vi "Main.vi"(11 "Module Admin":refnum<class "Delacor_lib_QMH_Module Admin.lvclass">) -> ()   [LabVIEW 2026, in "HMI.lvlib"]
doc: "This template is based off of the Queued Message Handler design pattern and the Queued Message Handler project template that ships with LabVIEW.\n\nThe main difference is that the queue is private to this module and communication between modules is performed via Broadcast and Request events.\n\nRequest events are wrapped in public API methods and are handled in the Event Handling Loop (EHL) of this VI. Any module can register for Broadcast events sent by this module. The EHL generates messages based on user interface actions.\n\nThe Message Handling Loop (MHL) processes messages generated by the EHL, or by other messages. The messages are string values, so new messages can be added easily to the Message Cases case structure in the MHL. Each message cluster can also provide an optional value for Message Data, which is a variant that can be converted to whatever message-specific data is required.\n_____\nBased on DQMH Dev Tools: Project Template 7.1.2.1547."
uses:
  HMI.lvlib
  <vilib>/Delacor/Delacor QMH/Libraries/Module Admin_class/Delacor_lib_QMH_Module Admin.lvclass
  Module Data--cluster.ctl
  <vilib>/Delacor/Delacor QMH/Libraries/Message Queue_class/Delacor_lib_QMH_Message Queue.lvclass/Delacor_lib_QMH_Message Queue.ctl
  Stop Argument--cluster.ctl
  <vilib>/Delacor/Delacor QMH/Libraries/Module Admin_class/Delacor_lib_QMH_Module Admin.lvclass/Delacor_lib_QMH_Module Admin.ctl
  <vilib>/Utility/miscctls.llb/LVPointTypeDef.ctl
  <vilib>/Delacor/Delacor QMH/Libraries/Message Queue_class/Delacor_lib_QMH_Enqueue Message (Single).vi
  <vilib>/Delacor/Delacor QMH/Libraries/Module Admin_class/Delacor_lib_QMH_Get External Launch.vi
  <vilib>/Delacor/Delacor QMH/Libraries/Message Queue_class/Delacor_lib_QMH_Message Queue.lvclass
  FT-818 CW Key Control/FT-818 CW Key Control.lvlib
  Plaintext to CW Sender/Plaintext to CW Sender.lvlib
panel:
  in  "CAT Rate":u32
  in  "Radio Comm Port":refnum<visa-resource-name>
  in  "Connect to FT-818":bool
  out "error out":errorcluster
  out "Status":string
  in  "Simulate MHL Error":bool
  in  "Simulate EHL Error":bool
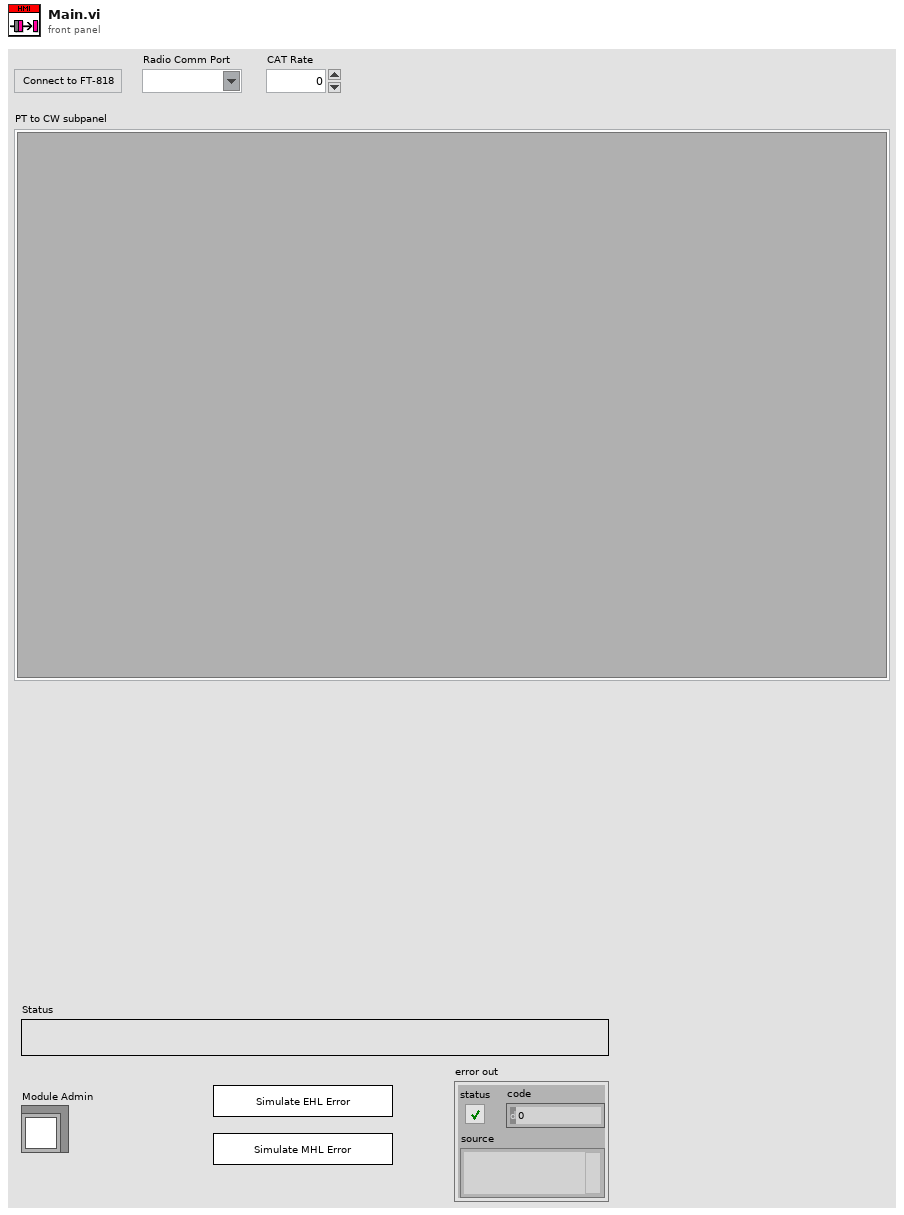
[diagram p1: front panel]
types:
  T1 = typedef "HMI.lvlib/Request Events--cluster.ctl" = cluster{"Stop Module":refnum<user-event>, "Show Panel":refnum<user-event>, "Hide Panel":refnum<user-event>, "Get Module Execution Status":refnum<user-event>, "Show Diagram":refnum<user-event>}
  T2 = typedef "FT-818 CW Key Control.lvlib/Broadcast Events--cluster.ctl" = cluster{"Module Did Init":refnum<user-event>, "Status Updated":refnum<user-event>, "Error Reported":refnum<user-event>, "Module Did Stop":refnum<user-event>, "Update Module Execution Status":refnum<user-event>}
  T3 = typedef "Plaintext to CW Sender.lvlib/Broadcast Events--cluster.ctl" = cluster{"Module Did Init":refnum<user-event>, "Status Updated":refnum<user-event>, "Error Reported":refnum<user-event>, "Module Did Stop":refnum<user-event>, "Update Module Execution Status":refnum<user-event>}
  T4 = typedef "HMI.lvlib/Module Data--cluster.ctl" = cluster{"Status":string}
  T5 = enum32{"invalid lock state", "Not Locked", "Locked (No Password)", "Password-protected"}
  T6 = typedef "HMI.lvlib/Stop Argument--cluster.ctl" = cluster{"Origin":string, "Exit via Stop Module Req?":bool, "Wait for Module to stop?":bool}
  T7 = typedef "LVPointTypeDef.ctl" = cluster{"Horizontal":i16, "Vertical":i16}
  T8 = enum32{"Invalid", "Standard", "Closed", "Hidden", "Minimized", "Maximized"}
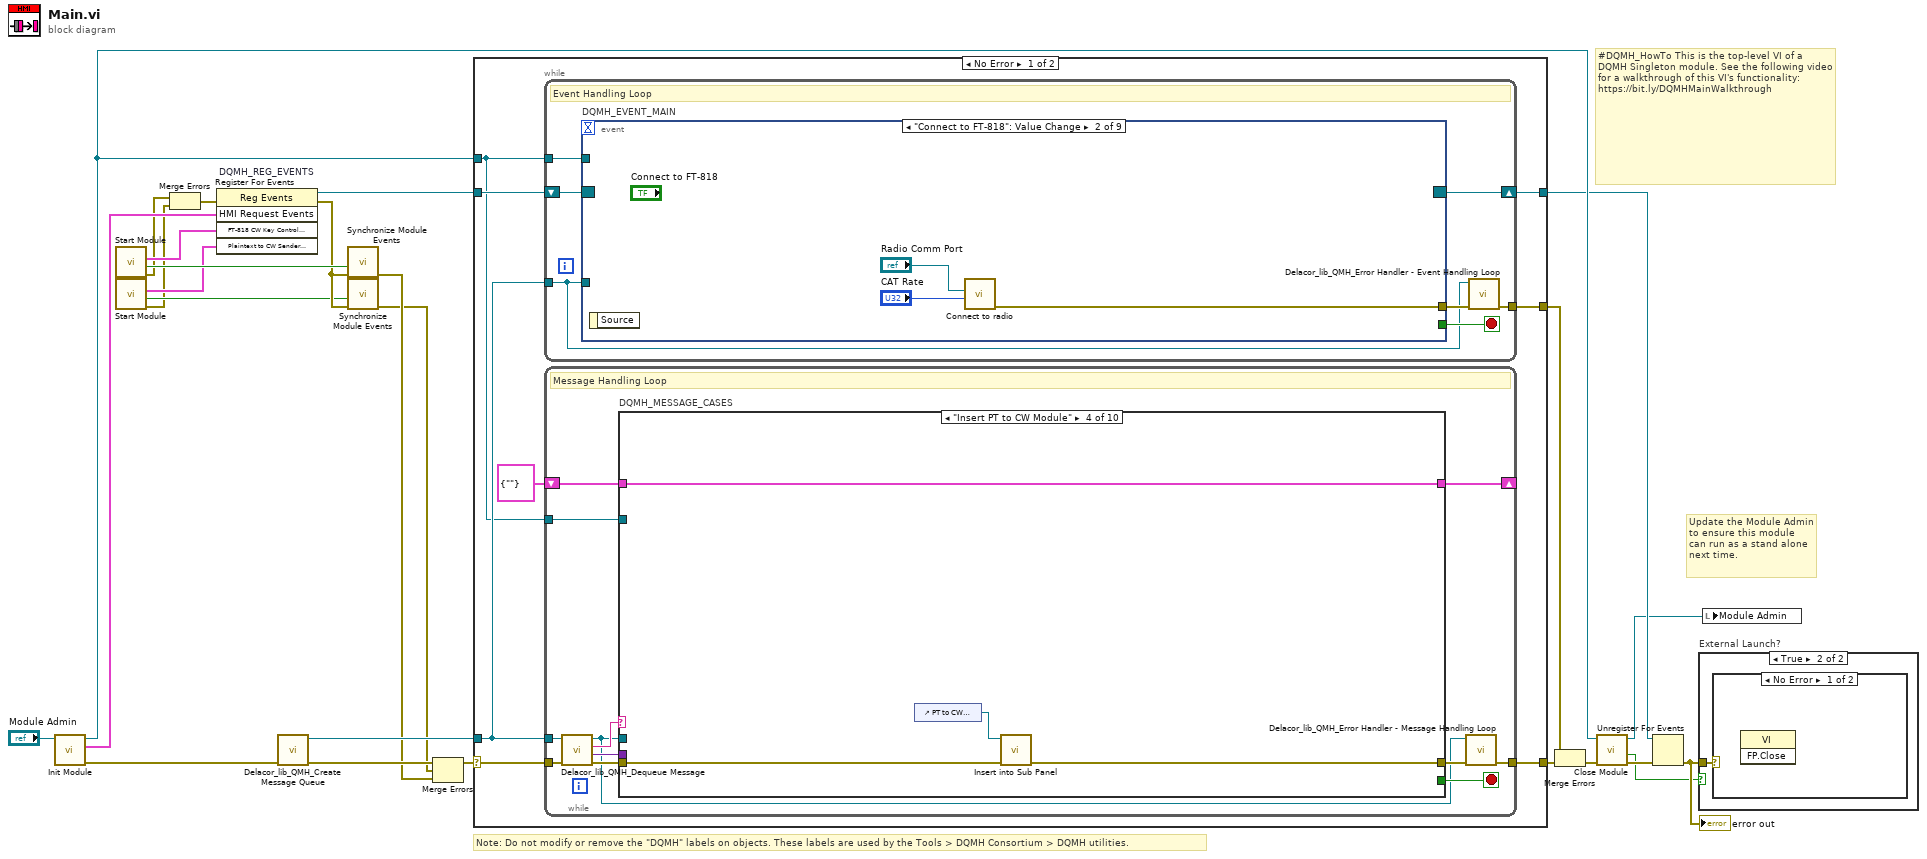
[diagram p0: block diagram]
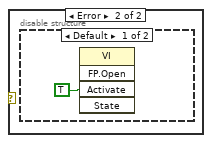
[diagram p3: hidden frame]
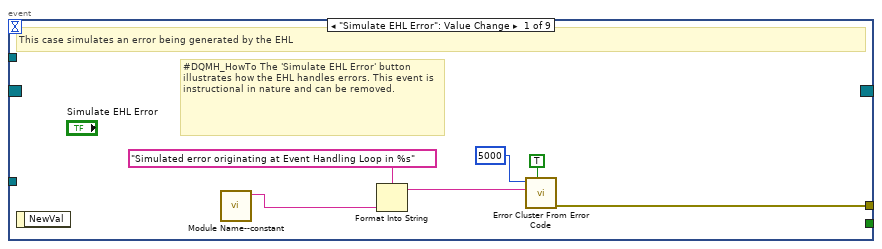
[diagram p5: hidden frame]
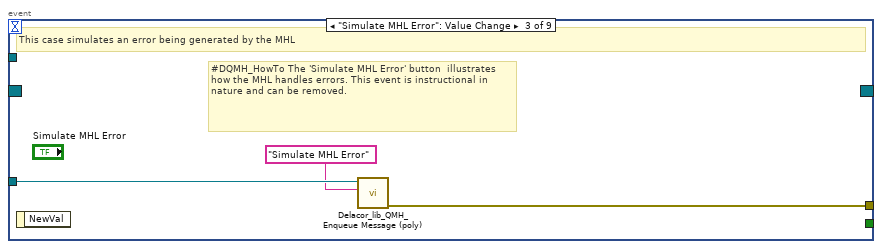
[diagram p6: hidden frame]
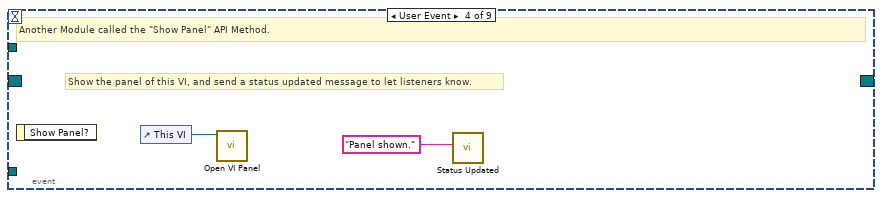
[diagram p7: hidden frame]
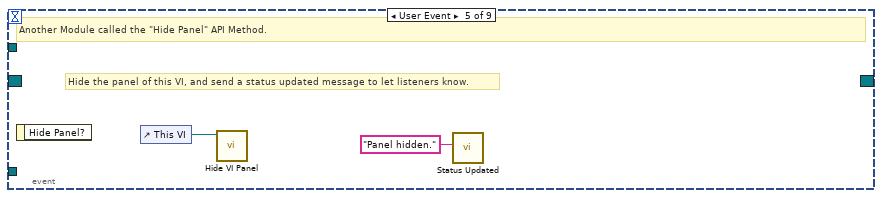
[diagram p8: hidden frame]
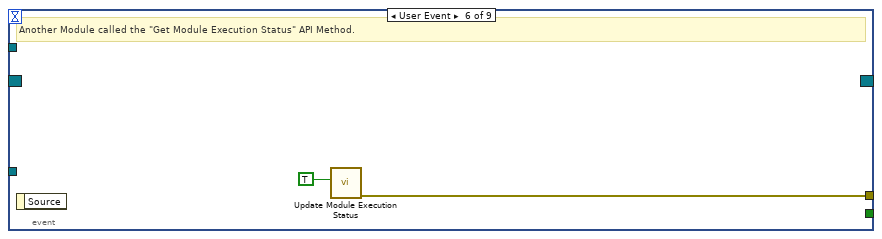
[diagram p9: hidden frame]
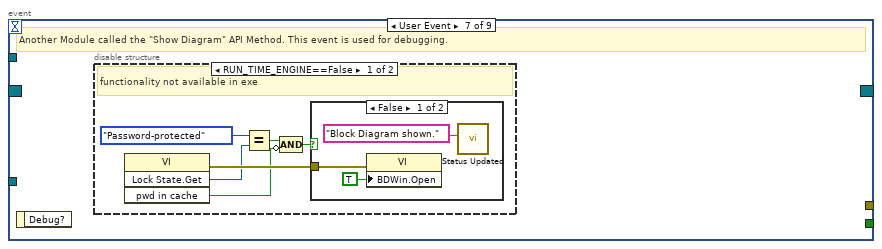
[diagram p10: hidden frame]
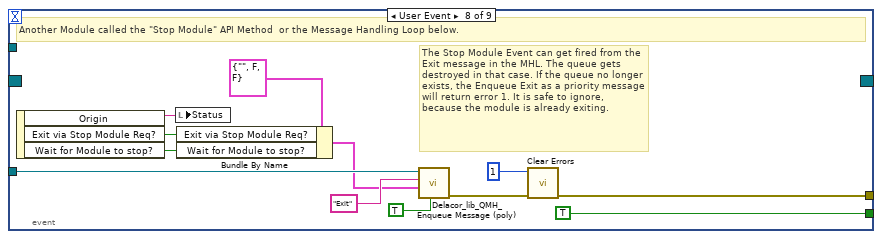
[diagram p13: hidden frame]
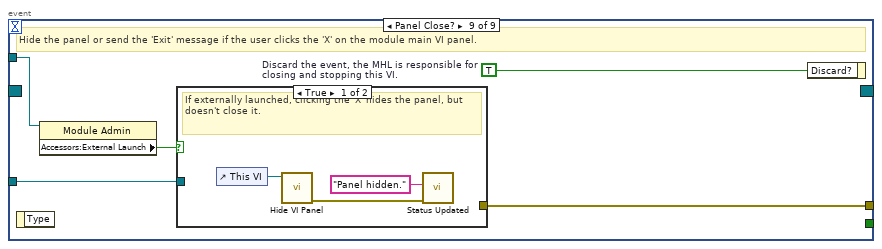
[diagram p14: hidden frame]
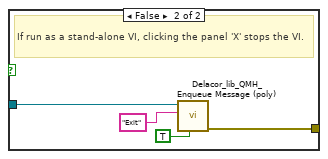
[diagram p15: hidden frame]
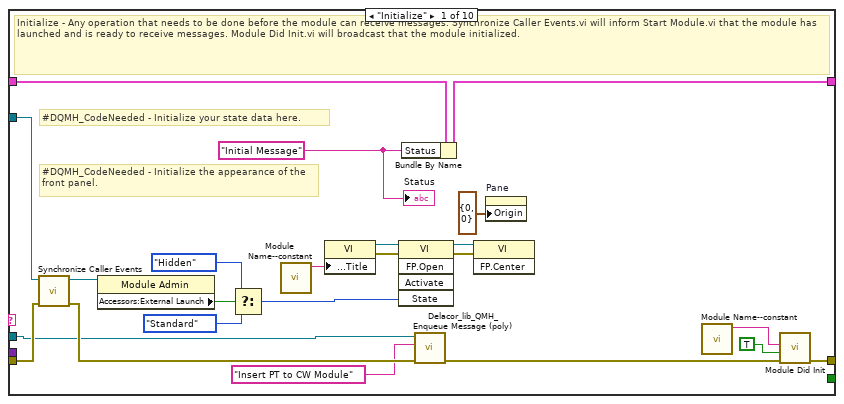
[diagram p16: hidden frame]
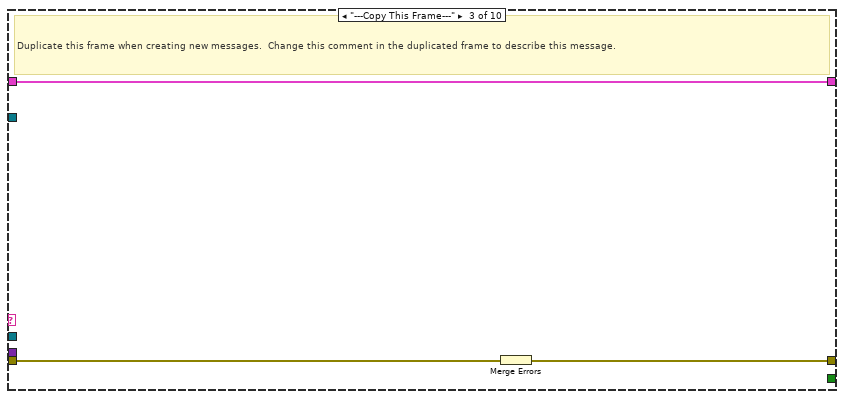
[diagram p18: hidden frame]
diagram:
  # "#DQMH_HowTo This is the top-level VI of a DQMH Singleton module. See the following video for a walkthrough of this VI's functionality: https://bit.ly/DQMHMainWalkthrough"
  # "Note: Do not modify or remove the \"DQMH\" labels on objects. These labels are used by the Tools > DQMH Consortium > DQMH utilities."
  # "Update the Module Admin to ensure this module can run as a stand alone next time."
  n1 = call "Init Module.vi"("Singleton Module Admin in"="Module Admin") -> ("error out"=w25:errorcluster, "HMI Request Events"=w15:T1, "Singleton Module Admin out"=w18:refnum<class "Delacor_lib_QMH_Module Admin.lvclass">)  [unwired: 8 in]
  n2 = call "Start Module.vi"() -> ("error out"=w3:errorcluster, "Wait for Event Sync?"=w9:bool, "FT-818 CW Key Control Broadcast Events"=w10:T2)  [unwired: 7 in, 2 out]
  n3 = call "Start Module.vi"() -> ("error out"=w2:errorcluster, "Wait for Event Sync?"=w4:bool, "Plaintext to CW Sender Broadcast Events"=w7:T3)  [unwired: 7 in, 2 out]
  n4 = Merge Errors(w3, w2) -> (w1:errorcluster)
  n5 = register-events "DQMH_REG_EVENTS"(error in=w1, w15, w10, w7) -> (reference out=w16:refnum<event-registration>, error out=w6:errorcluster)  [unwired: 1 in]
  n6 = call <vilib>:"Delacor_lib_QMH_Create Message Queue.vi"("error in"=w25) -> ("error out"=w20:errorcluster, "Message Queue"=w14:refnum<class "Delacor_lib_QMH_Message Queue.lvclass">)  [unwired: 9 in]
  n7 = call "Synchronize Module Events.vi"("error in"=w6, "Wait for Event Sync?"=w9) -> ("error out"=w8:errorcluster)  [unwired: 9 in]
  n8 = call "Synchronize Module Events.vi"("error in"=w6, "Wait for Event Sync?"=w4) -> ("error out"=w5:errorcluster)  [unwired: 9 in]
  n9 = Merge Errors(w20, w5, w8) -> (w19:errorcluster)
  n10 = case shown="No Error" w19 {
    selector: w19 -> [w32 w203]
    tunnel: [w34 w202] -> w26
    tunnel: [w31 w201] -> w17
    tunnel: w16 -> [w29 w201]
    tunnel: w14 -> [w28 w196]
    tunnel: [w33 _] -> w23
    tunnel: w18 -> [w27 w197]
    frame No Error {
      n11 = while {
        tunnel: w28 -> [w35]
        shift-right: [w38] -> w31
        shift-left: w29 -> [w39]
        tunnel: [w40] -> w33
        tunnel: w27 -> [w36]
        stop <- w37 stop-if-true
        # "Event Handling Loop"
        n12 = event "DQMH_EVENT_MAIN" shown="[1] \"Connect to FT-818\": Value Change" {
          selector: w39 -> [_ _ _ _ _ _ _ _ _]
          dyn-events: [_ _ _ _ _ _ _ _ _] -> w38
          timeout: _ -> [_ _ _ _ _ _ _ _ _]
          tunnel: [_ _ _ _ _ _ _ TRUE ("Discard?") _] -> w37
          tunnel: w35 -> [_ _ w52 _ _ _ _ w76 w83]
          tunnel: [w47 w50 w53 _ _ w59 _ w79 w85] -> w41
          tunnel: w36 -> [_ _ _ _ _ _ _ _ w82]
          event "Simulate EHL Error": Value Change {
            # "#DQMH_HowTo The 'Simulate EHL Error' button  illustrates how the EHL handles errors. This event is instructional in nature and can be removed."
            # "This case simulates an error being generated by the EHL"
            n13 = event-data() -> ()  [unwired: 1 in, 1 out]
            n14 = call "Module Name--constant.vi"() -> ("Module Name"=w44:string)  [unwired: 11 in]
            n15 = Format Into String(format string="Simulated error originating at Event Handling Loop in %s", w44) -> (resulting string=w45:string)  [unwired: 2 in, 1 out]
            n16 = call <vilib>:"Error Cluster From Error Code.vi"("show call chain? (False)"=TRUE, "error message (\"\")"=w45, "error code (0)"=5000) -> ("error out"=w47:errorcluster)  [unwired: 6 in]
          }
          event "Connect to FT-818": Value Change {
            n17 = event-data() -> ()  [unwired: 1 in, 1 out]
            n18 = call "Connect to radio.vi"("CAT Rate"="CAT Rate", "Radio Comm Port"="Radio Comm Port") -> ("error out"=w50:errorcluster)  [unwired: 7 in, 2 out]
          }
          event "Simulate MHL Error": Value Change {
            # "#DQMH_HowTo The 'Simulate MHL Error' button  illustrates how the MHL handles errors. This event is instructional in nature and can be removed."
            # "This case simulates an error being generated by the MHL"
            n19 = event-data() -> ()  [unwired: 1 in, 1 out]
            n20 = call-poly <vilib>:"Delacor_lib_QMH_Enqueue Message (poly).vi"("Message"="Simulate MHL Error", "Message Queue in"=w52) -> ("error out"=w53:errorcluster)  [unwired: 8 in, 1 out]
          }
          event User Event {
            # "Show the panel of this VI, and send a status updated message to let listeners know."
            # "Another Module called the \"Show Panel\" API Method."
            n21 = event-data() -> ()  [unwired: 1 in, 1 out]
            n22 = control-ref of="This VI"() -> (w55:refnum<vi>)
            n23 = call "Open VI Panel.vi"("VI"=w55) -> ()  [unwired: 10 in, 1 out]
            n24 = call "Status Updated.vi"("Status"="Panel shown." ("format string")) -> ()  [unwired: 10 in, 1 out]
          }
          event User Event {
            # "Hide the panel of this VI, and send a status updated message to let listeners know."
            # "Another Module called the \"Hide Panel\" API Method."
            n25 = event-data() -> ()  [unwired: 1 in, 1 out]
            n26 = control-ref of="This VI"() -> (w57:refnum<vi>)
            n27 = call "Hide VI Panel.vi"("VI"=w57) -> ()  [unwired: 10 in, 1 out]
            n28 = call "Status Updated.vi"("Status"="Panel hidden." ("format string")) -> ()  [unwired: 10 in, 1 out]
          }
          event User Event {
            # "Another Module called the \"Get Module Execution Status\" API Method."
            n29 = event-data() -> ()  [unwired: 1 in, 1 out]
            n30 = call "Update Module Execution Status.vi"("Running?"=TRUE) -> ("error out"=w59:errorcluster)  [unwired: 10 in]
          }
          event User Event {
            # "Another Module called the \"Show Diagram\" API Method. This event is used for debugging."
            n31 = event-data() -> ()  [unwired: 1 in, 1 out]
            n32 = disable-structure shown="RUN_TIME_ENGINE==False" {
              frame condition #0 (active) {
                # "functionality not available in exe"
                n33 = invoke on="Invoke Node" class="VI" method="Lock State.Get"() -> (error out=w65:errorcluster, "Get Lock State"=w64:T5, "pwd in cache"=w61:bool)  [unwired: 4 in, 1 out]
                n34 = Equal?(x=T5."Password-protected", y=w64) -> (x = y?=w62:bool)
                n35 = Compound Arithmetic op=AND(w62, invert w61) -> (w60:bool)
                n36 = case shown="False" w60 {
                  tunnel: w65 -> [w68 _]
                  frame False {
                    n37 = property on="Property Node" class="VI"(error in=w68, "BDWin.Open"=TRUE ("Block Diagram Window:Open")) -> ()  [unwired: 1 in, 2 out]
                    n38 = call "Status Updated.vi"("Status"="Block Diagram shown." ("format string")) -> ()  [unwired: 10 in, 1 out]
                  }
                  frame True {
                    # "Password-protected VI, and the password is not in the cache. Do not show the diagram."
                  }
                }
              }
              frame condition #1 {
              }
            }
          }
          event User Event {
            # "The Stop Module Event can get fired from the Exit message in the MHL. The queue gets destroyed in that case. If the queue no longer exists, the Enqueue Exit as a priority message will return error 1. It is safe to ignore, because the module is already exiting."
            # "Another Module called the \"Stop Module\" API Method  or the Message Handling Loop below."
            n39 = event-data() -> ("Origin"=w75:string, "Exit via Stop Module Req?"=w71:bool, "Wait for Module to stop?"=w70:bool)  [unwired: 1 in]
            n40 = local write "Status"(w75) -> ()
            n41 = Bundle By Name(cluster=T6 {"Origin"="", "Exit via Stop Module Req?"=FALSE, "Wait for Module to stop?"=FALSE} ("Stop Argument"), "Exit via Stop Module Req?"=w71, "Wait for Module to stop?"=w70) -> (w69:T6)
            n42 = call-poly <vilib>:"Delacor_lib_QMH_Enqueue Message (poly).vi"("Priority Message? (F)"=TRUE, "Message Data"=w69, "Message"="Exit", "Message Queue in"=w76) -> ("error out"=w80:errorcluster)  [unwired: 6 in, 1 out]
            n43 = call <vilib>:"Clear Errors.vi"("error in (no error)"=w80, "specific error code to clear (0: all)"=1) -> ("error out"=w79:errorcluster)  [unwired: 4 in, 1 out]
          }
          event Panel Close? {
            w84 = TRUE  # Discard the event, the MHL is responsible for closing and stopping this VI.
            # "Hide the panel or send the 'Exit' message if the user clicks the 'X' on the module main VI panel."
            n44 = event-data() -> ()  [unwired: 1 in, 1 out]
            n45 = property on="Property Node" class="Module Admin"(reference=w82) -> ("Accessors:External Launch"=w81:bool)  [unwired: 1 in, 2 out]
            n46 = case shown="True" w81 {
              tunnel: w83 -> [_ w91]
              tunnel: [_ w92] -> w85
              frame True {
                # "If externally launched, clicking the 'X' hides the panel, but doesn't close it."
                n47 = control-ref of="This VI"() -> (w88:refnum<vi>)
                n48 = call "Hide VI Panel.vi"("VI"=w88) -> ("error out"=w86:errorcluster)  [unwired: 10 in]
                n49 = call "Status Updated.vi"("error in"=w86, "Status"="Panel hidden." ("format string")) -> ()  [unwired: 9 in, 1 out]
              }
              frame False {
                # "If run as a stand-alone VI, clicking the panel 'X' stops the VI."
                n50 = call-poly <vilib>:"Delacor_lib_QMH_Enqueue Message (poly).vi"("Priority Message? (F)"=TRUE, "Message"="Exit", "Message Queue in"=w91) -> ("error out"=w92:errorcluster)  [unwired: 7 in, 1 out]
              }
            }
            n51 = event-data ("Event Filter Node")("Discard?"=w84) -> ()  [unwired: 1 in, 1 out]
          }
        }
        n52 = call-dynamic "Delacor_lib_QMH_Error Handler - Event Handling Loop.vi"("error in"=w41, "Message Queue in"=w35) -> ("dup error in"=w40:errorcluster)  [unwired: 8 in, 1 out]
      }
      n53 = while {
        tunnel: w28 -> [w93]
        shift-right: [w101] -> _
        shift-left: T4 {"Status"=""} ("Data Cluster") -> [w102]
        tunnel: w32 -> [w104]
        tunnel: [w96] -> w34
        tunnel: w27 -> [w97]
        stop <- w100 stop-if-true
        # "Message Handling Loop"
        n54 = call-dynamic "Delacor_lib_QMH_Dequeue Message.vi"("error in"=w104, "Message Queue in"=w93) -> ("error out"=w103:errorcluster, "Message Data"=w98:variant, "Message"=w99:string, "Message Queue out"=w94:refnum<class "Delacor_lib_QMH_Message Queue.lvclass">)  [unwired: 6 in]
        n55 = case "DQMH_MESSAGE_CASES" shown="\"Insert PT to CW Module\"" w99 {
          selector: w99 -> [_ _ _ _ _ _ _ _ _ w191]
          tunnel: w94 -> [w106 _ _ _ _ _ _ w153 w179 _]
          tunnel: w103 -> [w125 w129 w132 w135 w138 w140 w149 w160 w185 w194]
          tunnel: [w123 w129 w131 w134 w138 w140 w148 w156 w180 w195] -> w95
          tunnel: w102 -> [w114 w128 w130 w136 w137 w139 w146 w155 w178 w192]
          tunnel: [w113 w128 w130 w136 w137 w139 w146 w155 w178 w192] -> w101
          tunnel: [_ _ _ _ _ _ _ _ w177 _] -> w100
          tunnel: w98 -> [_ _ _ _ _ _ _ w154 w176 _]
          tunnel: w97 -> [w115 _ _ _ _ _ _ w152 w171 _]
          frame "Initialize" {
            w109 = "Initial Message" ("Initial Message")
            # "#DQMH_CodeNeeded - Initialize the appearance of the front panel."
            # "#DQMH_CodeNeeded - Initialize your state data here."
            # "Initialize - Any operation that needs to be done before the module can receive messages. Synchronize Caller Events.vi will inform Start Module.vi that the module has launched and is ready to receive messages. Module Did Init.vi will broadcast that the module initialized."
            n56 = call "Synchronize Caller Events.vi"("error in"=w125, "Singleton Module Admin in"=w115) -> ("error out"=w124:errorcluster, "Singleton Module Admin out"=w110:refnum<class "Delacor_lib_QMH_Module Admin.lvclass">)  [unwired: 8 in]
            n57 = property on="Property Node" class="Module Admin"(reference=w110) -> ("Accessors:External Launch"=w119:bool)  [unwired: 1 in, 2 out]
            n58 = Select(t=T8."Hidden" ("State"), s=w119, f=T8."Standard" ("State")) -> (s? t:f=w116:T8)
            n59 = call "Module Name--constant.vi"() -> ("Module Name"=w122:string)  [unwired: 11 in]
            n60 = property on="Property Node" class="VI"("Front Panel.Title"=w122) -> (reference out=w121:refnum<vi>, error out=w127:errorcluster)  [unwired: 2 in]
            n61 = invoke on="Invoke Node" class="VI" method="FP.Open"(reference=w121, error in=w127, "State"=w116) -> (reference out=w120:refnum<vi>, error out=w126:errorcluster)  [unwired: 2 in, 3 out]
            n62 = Bundle By Name(cluster=w114, "Status"=w109) -> (w113:T4)
            n63 = call-poly <vilib>:"Delacor_lib_QMH_Enqueue Message (poly).vi"("error in"=w124, "Message"="Insert PT to CW Module", "Message Queue in"=w106) -> ("error out"=w107:errorcluster)  [unwired: 7 in, 1 out]
            n64 = invoke on="Invoke Node" class="VI" method="FP.Center"(reference=w120, error in=w126) -> ()  [unwired: 1 in, 3 out]
            n65 = property on="Pane" class="Pane"("Origin"=T7 {"Horizontal"=0, "Vertical"=0}) -> ()  [unwired: 2 in, 2 out]
            n66 = call "Module Name--constant.vi"() -> ("Module Name"=w111:string)  [unwired: 11 in]
            n67 = call "Module Did Init.vi"("error in"=w107, "Initialized?"=TRUE, "Origin"=w111) -> ("error out"=w123:errorcluster)  [unwired: 8 in]
            "Status" <- w109
          }
          frame "---Module Specific---" {
            # "Separator -- The following cases handle messages specific to this Module."
          }
          frame "---Copy This Frame---" {
            # "Duplicate this frame when creating new messages.  Change this comment in the duplicated frame to describe this message."
            n68 = Merge Errors(w132) -> (w131:errorcluster)
          }
          frame "Insert PT to CW Module" {
            n69 = control-ref of="PT to CW subpanel"() -> (w133:refnum<vi>)
            n70 = call "Insert into Sub Panel.vi"("error in (no error)"=w135, "Sub Panel Reference"=w133) -> ("error out"=w134:errorcluster)  [unwired: 8 in, 1 out]
          }
          frame "Start FT-818 Module" {
          }
          frame "---Exit and Error Handling---" {
            # "Separator - The following cases handle errors and exit messages."
          }
          frame "Simulate MHL Error" {
            # "#DQMH_HowTo The 'Simulate MHL Error' button  illustrates how the MHL handles errors. This event is instructional in nature and can be removed."
            # "Simulate an error occurring at the MHL"
            n71 = call "Module Name--constant.vi"() -> ("Module Name"=w142:string)  [unwired: 11 in]
            n72 = Format Into String(format string="Simulated error originating at Message Handling Loop in %s", w142) -> (resulting string=w143:string)  [unwired: 2 in, 1 out]
            n73 = call <vilib>:"Error Cluster From Error Code.vi"("show call chain? (False)"=TRUE, "error message (\"\")"=w143, "error code (0)"=5001) -> ("error out"=w147:errorcluster)  [unwired: 6 in]
            n74 = Merge Errors(w149, w147) -> (w148:errorcluster)
          }
          frame "Error" {
            # "#DQMH_CodeRecommended - If the module is running in standalone mode (External Launch = FALSE), this code will pop up an error dialog and call the 'Exit' message if an error occurs. Add more fine-grained error management here."
            # "Error - Check the error message data and respond accordingly. This message is sent by the \"Error Handler\" VIs at the end of each loop in this application."
            n75 = property on="Property Node" class="Module Admin"(reference=w152) -> ("Accessors:External Launch"=w151:bool)  [unwired: 1 in, 2 out]
            n76 = Variant To Data(error in=w160, type=errorcluster {"status"=FALSE, "code"=0, "source"=""} ("error constant"), Variant=w154) -> (data=w150:errorcluster, error out=w158:errorcluster)
            n77 = local write "error out"(w150) -> ()
            n78 = call "Error Reported.vi"("Error"=w150) -> ()  [unwired: 10 in, 1 out]
            n79 = case shown="False" w151 {
              tunnel: [w165 _] -> w157
              tunnel: w153 -> [w163 _]
              tunnel: w150 -> [w164 _]
              frame False {
                n80 = disable-structure shown="Default" {
                  disable-tunnel: w164 -> [w166 _]
                  frame condition #0 (active) {
                    # "If the module is running standalone, then pop up an error dialog and call the \"Exit\" message."
                    n81 = call <vilib>:"Simple Error Handler.vi"("error in (no error)"=w166) -> ()  [unwired: 4 in, 5 out]
                  }
                  frame condition #1 {
                    # "To prevent the Simple Error Handler VI from being loaded (e.g. when deploying to a Real-Time target), add the Conditional Disable Symbol \"DQMH_Disable_SEH\" to your project and set it to TRUE."
                  }
                }
                n82 = call-poly <vilib>:"Delacor_lib_QMH_Enqueue Message (poly).vi"("Priority Message? (F)"=TRUE, "Message"="Exit", "Message Queue in"=w163) -> ("error out"=w165:errorcluster)  [unwired: 7 in, 1 out]
              }
              frame True {
                # "If the module was launched externally, calling the Error Reported broadcast VI is the only action performed by the \"Error\" message. The module's caller can then process the error appropriately."
              }
            }
            n83 = Merge Errors(w158, w157) -> (w156:errorcluster)
          }
          frame "Exit" {
            w175 = 91  # 91: not all Exit messages will have an argument
            w177 = TRUE  # Stop the VI
            # "Release the message queue reference"
            # "#DQMH_CodeNeeded - Add any required cleanup code here."
            # "Exit - Exit the application."
            n84 = Variant To Data(error in=w185, type=T6 {"Origin"="", "Exit via Stop Module Req?"=FALSE, "Wait for Module to stop?"=FALSE} ("Stop Argument"), Variant=w176) -> (data=w173:T6, error out=w182:errorcluster)
            n85 = call <vilib>:"Clear Errors.vi"("error in (no error)"=w182, "specific error code to clear (0: all)"=w175) -> ("error out"=w184:errorcluster)  [unwired: 4 in, 1 out]
            n86 = control-ref of="This VI"() -> (w172:refnum<vi>)
            n87 = call-dynamic "Delacor_lib_QMH_Release Message Queue.vi"("error in"=w184, "Message Queue"=w179) -> ("error out"=w183:errorcluster)  [unwired: 9 in]
            n88 = call "Handle Exit.vi"("Stop Argument"=w173, "Admin in"=w171, "VI reference"=w172) -> ("error out"=w181:errorcluster)  [unwired: 7 in, 1 out]
            n89 = control-ref of="PT to CW subpanel"() -> (w169:refnum<vi>)
            n90 = invoke class="SubPnl" method="Remove VI"(reference=w169) -> (error out=w168:errorcluster)  [unwired: 2 in, 2 out]
            n91 = call "Stop Module.vi"("error in"=w168) -> ("error out"=w167:errorcluster)  [unwired: 10 in]
            n92 = call "Stop Module.vi"() -> ("error out"=w170:errorcluster)  [unwired: 11 in]
            n93 = Merge Errors(w167, w170, w183, w181) -> (w180:errorcluster)
            n94 = call "Error Reported.vi"("Error"=w180) -> ()  [unwired: 10 in, 1 out]
          }
          frame Default {
            # "'Default' case only runs if there is a message that isn't defined in any of the other cases.  Output a programming error."
            n95 = call "Module Name--constant.vi"() -> ("Module Name"=w190:string)  [unwired: 11 in]
            n96 = Format Into String(format string="The invalid message string \"%s\" was received in the Message Handling Loop for module \"%s\".", w191, w190) -> (resulting string=w186:string)  [unwired: 2 in, 1 out]
            n97 = call <vilib>:"Error Cluster From Error Code.vi"("show call chain? (False)"=TRUE, "error message (\"\")"=w186, "error code (0)"=1) -> ("error out"=w193:errorcluster)  [unwired: 6 in]
            n98 = Merge Errors(w194, w193) -> (w195:errorcluster)
          }
        }
        n99 = call-dynamic "Delacor_lib_QMH_Error Handler - Message Handling Loop.vi"("error in"=w95, "Message Queue in"=w94) -> ("dup error in"=w96:errorcluster)  [unwired: 8 in, 1 out]
      }
    }
    frame Error {
      # "Synchronize Caller Events.vi will inform Start Module.vi that the module has launched and will let the code calling Start Module.vi register for broadcasts and would permit the caller receive the broadcast that an error occurred at launch time."
      n100 = call-dynamic "Delacor_lib_QMH_Release Message Queue.vi"("error in"=w203, "Message Queue"=w196) -> ("error out"=w202:errorcluster)  [unwired: 9 in]
      n101 = call "Synchronize Caller Events.vi"("Singleton Module Admin in"=w197) -> ("error out"=w204:errorcluster)  [unwired: 9 in, 1 out]
      n102 = call "Module Name--constant.vi"() -> ("Module Name"=w200:string)  [unwired: 11 in]
      n103 = Format Into String(format string="An error occurred during initialization. %s is no longer running.", w200) -> (resulting string=w198:string)  [unwired: 2 in, 1 out]
      n104 = Merge Errors(w202, w204) -> (w205:errorcluster)
      n105 = call "Error Reported.vi"("Additional Information"=w198, "Error"=w205) -> ()  [unwired: 9 in, 1 out]
    }
  }
  n106 = Merge Errors(w23, w26) -> (w22:errorcluster)
  n107 = call "Close Module.vi"("error in"=w22, "Module Admin in"=w18) -> ("error out"=w24:errorcluster, "External Launch"=w11:bool, "Module Admin out"=w12:refnum<class "Delacor_lib_QMH_Module Admin.lvclass">)  [unwired: 7 in]
  n108 = Unregister For Events(event registration refnum=w17, error in=w24) -> (error out=w21:errorcluster)
  "error out" <- w21
  n109 = case "External Launch?" shown="True" w11 {
    tunnel: w21 -> [_ w206]
    frame False {
    }
    frame True {
      n110 = case shown="No Error" w206 {
        frame No Error {
          n111 = invoke on="Invoke Node" class="VI" method="FP.Close"() -> ()  [unwired: 3 in, 3 out]
        }
        frame Error {
          n112 = disable-structure shown="Default" {
            frame condition #0 (active) {
              n113 = invoke class="VI" method="FP.Open"("Activate"=TRUE ("Activate?")) -> ()  [unwired: 4 in, 5 out]
            }
            frame condition #1 {
              # "Don't show panel on error if running inside a built EXE."
            }
          }
        }
      }
    }
  }
  n114 = local write "Module Admin"(w12) -> ()
